vi "Unregister (JSON).vi"(7 "Options":string, 8 "error in (no error)":errorcluster, 9 "Time out ms (1000)":i32=1000, 10 "URI":string, 11 "WAMP Client in":refnum<class "WAMP Client.lvclass">) -> (0 "error out":errorcluster, 3 "WAMP Client out":refnum<class "WAMP Client.lvclass">, 5 "WAMP Error":T1={"URI"="", "Arguments Payload"="", "ArgumentKw Payload"="{}", "Details"="{}"})   [LabVIEW 2020, in "wamplv.lvlib" / "WAMP Client.lvclass"]
uses:
  WAMP Client.lvclass
  WAMP Client.lvclass/WAMP Client.ctl
  621c6210-80ea-441c-aa52-19dc047a6863.vi
  TypeDefs/Error or abort detail (JSON).ctl
  wamplv.lvlib
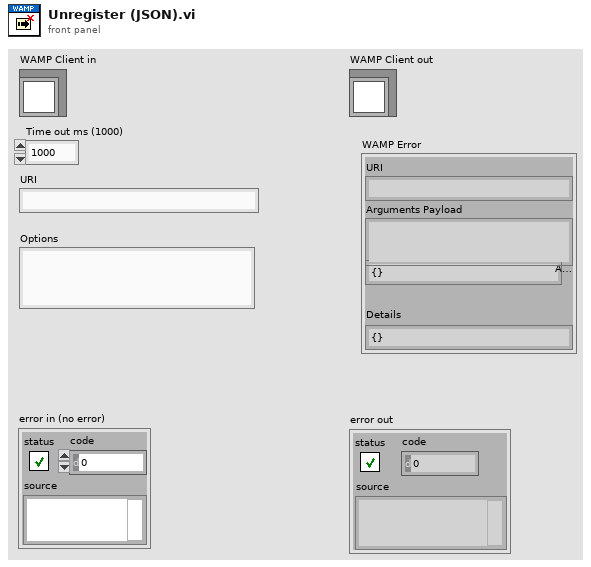
[diagram p1: front panel]
types:
  T1 = typedef "wamplv.lvlib/Error or abort detail (JSON).ctl" = cluster{"URI":string, "Arguments Payload":string, "ArgumentKw Payload":string, "Details":string}
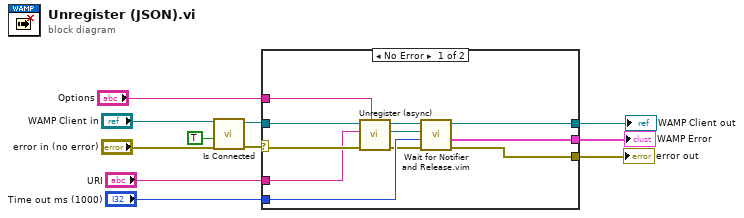
[diagram p0: block diagram]
diagram:
  n1 = call "Is Connected.vi"("error in"="error in (no error)", "Raise error if not connected"=TRUE, "WAMP Client in"="WAMP Client in") -> ("error out"=w4:errorcluster, "WAMP Client out"=w2:refnum<class "WAMP Client.lvclass">)  [unwired: 6 in, 1 out]
  n2 = case shown="No Error" w4 {
    selector: w4 -> [w22 w24]
    tunnel: [w19 w24] -> w11
    tunnel: [w17 w23] -> w10
    tunnel: w2 -> [w12 w23]
    tunnel: "Time out ms (1000)" -> [w20 _]
    tunnel: "URI" -> [w21 _]
    tunnel: [w18 _] -> w8
    tunnel: "Options" -> [w16 _]
    frame No Error {
      n3 = call "Unregister (async).vi"("Options"=w16, "error in (no error)"=w22, "Endpoint URI"=w21, "WAMP Client in"=w12) -> ("error out"=w13:errorcluster, "notifier out"=w15:refnum<notifier>, "WAMP Client out"=w14:refnum<class "WAMP Client.lvclass">)  [unwired: 5 in]
      n4 = call "Wait for Notifier and Release.vim"("error in (no error)"=w13, "timeout in ms (0)"=w20, "Notifier in"=w15, "WAMP Client in"=w14) -> ("error out"=w19:errorcluster, "WAMP Error"=w18:T1, "WAMP Client out"=w17:refnum<class "WAMP Client.lvclass">)  [unwired: 4 in, 1 out]
    }
    frame Error {
    }
  }
  "error out" <- w11
  "WAMP Client out" <- w10
  "WAMP Error" <- w8
